vi "Tx Async.vi"(8 "error in (no error)":errorcluster, 10 "Dispatcher Interface in":refnum<class "Dispatcher Interface.lvclass">, 11 "Plugin in":refnum<class "Plugin.lvclass">) -> (0 "error out":errorcluster, 2 "Dispatcher Interface out":refnum<class "Dispatcher Interface.lvclass">, 3 "Plugin out":refnum<class "Plugin.lvclass">)   [LabVIEW 2017, in "DSF Core.lvlib" / "Plugin.lvclass"]
uses:
  Plugin.lvclass
  Interface/Dispatcher/Dispatcher Interface.lvclass
  Plugin.lvclass/Plugin.ctl
  Interface/Dispatcher/Command.ctl
  Transfer Group/Transfer Group.lvclass/Transfer Group.ctl
  Transfer Group/Transfer Group.lvclass
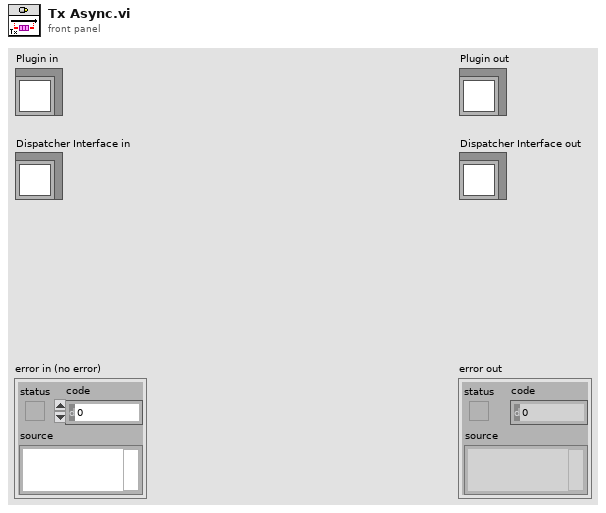
[diagram p1: front panel]
types:
  T1 = typedef "DSF Core.lvlib/Dispatcher Interface.lvclass/Command.ctl" = enum8{"Idle", "Start", "Rx", "Tx", "Set Inline Buffer", "Shutdown", "Error"}
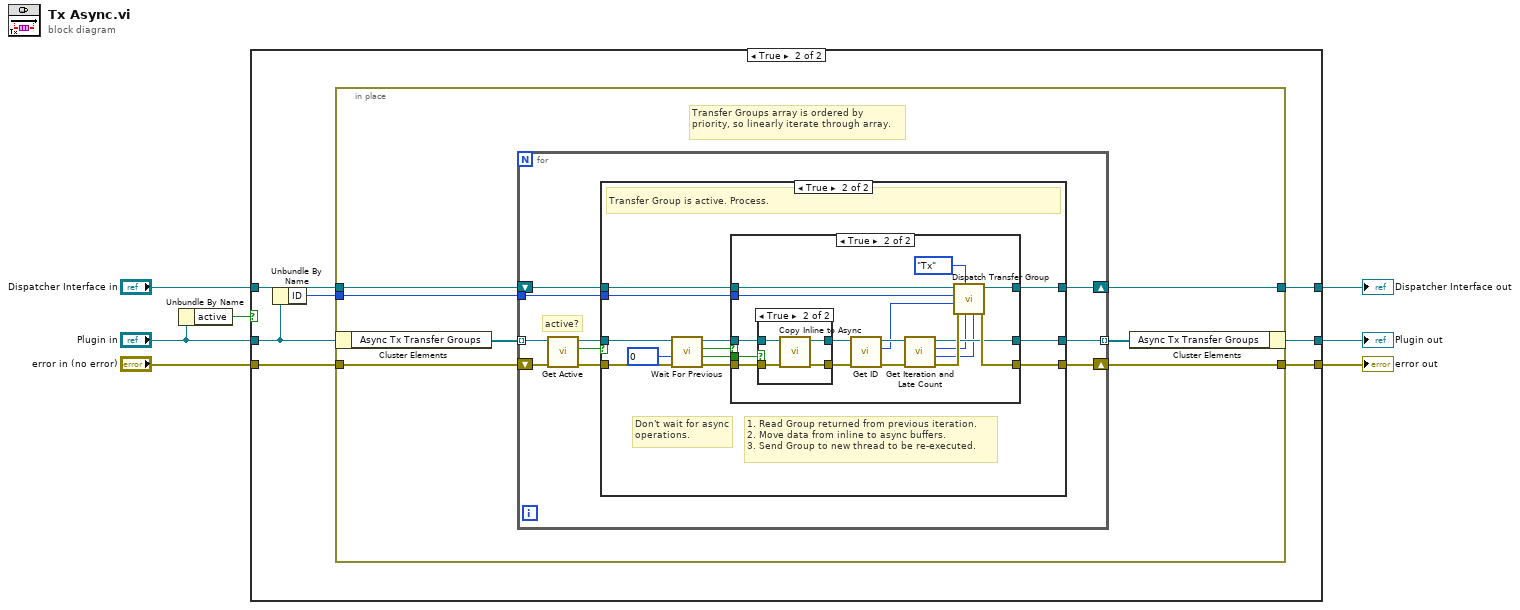
[diagram p0: block diagram]
diagram:
  n1 = Unbundle By Name("Plugin in") -> ("active"=w1:bool)
  n2 = case shown="True" w1 {
    tunnel: "error in (no error)" -> [w8 w17]
    tunnel: [w8 w16] -> w6
    tunnel: [w9 w15] -> w5
    tunnel: "Plugin in" -> [w9 w11]
    tunnel: "Dispatcher Interface in" -> [w10 w14]
    tunnel: [w10 w13] -> w3
    frame False {
    }
    frame True {
      n3 = Unbundle By Name(w11) -> ("ID"=w12:i32)
      n4 = in-place {
        in-place-border: w17 -> [w24]
        in-place-border: [w23] -> w16
        in-place-border: w12 -> [w20]
        in-place-border: w14 -> [w19]
        in-place-border: [w18] -> w13
        # "Transfer Groups array is ordered by priority, so linearly iterate through array."
        n5 = in-place-cluster #1(w11) -> ("Async Tx Transfer Groups"=w22:refnum<class "Transfer Group.lvclass">[])
        n6 = for {
          tunnel: w22 -> [w27] mode=indexing
          shift-right: [w31] -> w23
          shift-left: w24 -> [w33]
          tunnel: [w32] -> w21 mode=indexing
          tunnel: w20 -> [w30]
          shift-right: [w28] -> w18
          shift-left: w19 -> [w29]
          # "active?"
          n7 = call "Get Active.vi"("Transfer Group in"=w27) -> ("active"=w25:bool, "Transfer Group out"=w26:refnum<class "Transfer Group.lvclass">)  [unwired: 9 in]
          n8 = case shown="True" w25 {
            tunnel: [w36 w38] -> w31
            tunnel: w33 -> [w36 w43]
            tunnel: w26 -> [w35 w44]
            tunnel: [w35 w39] -> w32
            tunnel: w30 -> [_ w40]
            tunnel: w29 -> [w34 w42]
            tunnel: [w34 w41] -> w28
            frame False {
              # "Transfer Group is not active. Skip."
            }
            frame True {
              # "Don't wait for async operations."
              # "1. Read Group returned from previous iteration.\n2. Move data from inline to async buffers.\n3. Send Group to new thread to be re-executed."
              # "Transfer Group is active. Process."
              n9 = call "Wait For Previous.vi"("error in (no error)"=w43, "timeout in ms (0)"=0, "Transfer Group in"=w44) -> ("error out"=w48:errorcluster, "move data"=w37:bool, "ready"=w47:bool, "Transfer Group out"=w46:refnum<class "Transfer Group.lvclass">)  [unwired: 5 in]
              n10 = case shown="True" w47 {
                tunnel: w46 -> [w51 w56]
                tunnel: [w51 w61] -> w39
                tunnel: [w50 w62] -> w38
                tunnel: w48 -> [w50 w55]
                tunnel: [w49 w59] -> w41
                tunnel: w42 -> [w49 w58]
                tunnel: w40 -> [_ w57]
                tunnel: w37 -> [_ w53]
                frame False {
                }
                frame True {
                  n11 = case shown="True" w53 {
                    tunnel: w56 -> [w68 w73]
                    tunnel: w55 -> [w69 w72]
                    tunnel: [w68 w71] -> w52
                    tunnel: [w69 w70] -> w66
                    frame False {
                    }
                    frame True {
                      n12 = call "Copy Inline to Async.vi"("error in (no error)"=w72, "Transfer Group in"=w73) -> ("error out"=w70:errorcluster, "Transfer Group out"=w71:refnum<class "Transfer Group.lvclass">)  [unwired: 8 in]
                    }
                  }
                  n13 = call "Get ID.vi"("Transfer Group in"=w52) -> ("id"=w65:i32, "Transfer Group out"=w67:refnum<class "Transfer Group.lvclass">)  [unwired: 9 in]
                  n14 = call "Get Iteration and Late Count.vi"("error in (no error)"=w66, "Transfer Group in"=w67) -> ("error out"=w64:errorcluster, "late count"=w54:i32, "iteration"=w60:u64, "Transfer Group out"=w61:refnum<class "Transfer Group.lvclass">)  [unwired: 6 in]
                  n15 = call "Dispatch Transfer Group.vi"("Late Count"=w54, "Iteration"=w60, "command"=Command."Tx", "error in (no error)"=w64, "Transfer Group ID"=w65, "Plugin ID"=w57, "Dispatcher Interface in"=w58) -> ("error out"=w62:errorcluster, "Dispatcher Interface out"=w59:refnum<class "Dispatcher Interface.lvclass">)  [unwired: 3 in]
                }
              }
            }
          }
        }
        n16 = in-place-cluster #1("Async Tx Transfer Groups"=w21) -> (w15:refnum<class "Plugin.lvclass">)
      }
    }
  }
  "error out" <- w6
  "Plugin out" <- w5
  "Dispatcher Interface out" <- w3
